vi "Amp_PS_onoff.vi"(2 "error in (no error)":errorcluster, 3 "On/Off Control":string(combo), 4 "delay before read (ms)":u32=500, 5 "Amp PS address":refnum<visa-resource-name>) -> (0 "error out":errorcluster, 1 "status":bool)   [LabVIEW 2019]
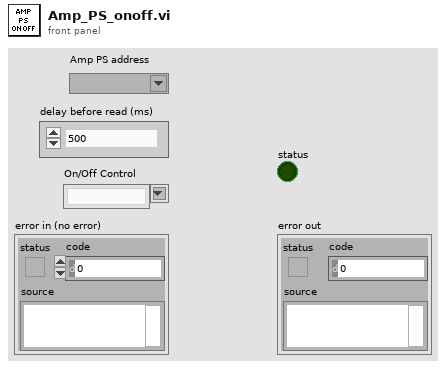
[diagram p1: front panel]
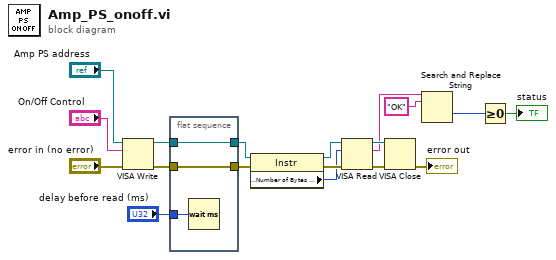
[diagram p0: block diagram]
diagram:
  n1 = VISA Write(VISA resource name="Amp PS address", write buffer="On/Off Control", error in (no error)="error in (no error)") -> (VISA resource name out=w14:refnum<visa-resource-name>, error out=w16:errorcluster)  [unwired: 1 out]
  n2 = flat-sequence {
    tunnel: w16 -> [w20]
    tunnel: [w20] -> w15
    tunnel: w14 -> [w19]
    tunnel: [w19] -> w13
    tunnel: "delay before read (ms)" -> [w21]
    frame #0 {
      n3 = Wait (ms)(milliseconds to wait=w21) -> ()  [unwired: 1 out]
    }
  }
  n4 = property class="Instr"(reference=w13, error in=w15) -> (reference out=w12:refnum<visa-resource-name>, error out=w11:errorcluster, "Serial Settings:Number of Bytes at Serial Port"=w10:u32)
  n5 = VISA Read(VISA resource name=w12, byte count=w10, error in (no error)=w11) -> (VISA resource name out=w17:refnum<visa-resource-name>, read buffer=w5:string, error out=w18:errorcluster)  [unwired: 1 out]
  n6 = VISA Close(VISA resource name=w17, error in (no error)=w18) -> (error out=→"error out":errorcluster)
  n7 = Search and Replace String(input string=w5, search string="OK" ("true string")) -> (offset past replacement=w3:i32)  [unwired: 6 in, 3 out]
  n8 = Greater Or Equal To 0?(x=w3) -> (x >= 0?=→"status":bool)
